vi "Set VRISE.vi"(0 "VISA resource name":refnum<visa-resource-name>, 2 "cluster":cluster{bool, bool, bool, bool}, 5 "error in (no error)":errorcluster) -> (14 "VISA resource name out":refnum<visa-resource-name>, 15 "concatenated string":string, 18 "?":T1 {"Channel 1" format="%#_6e"; "Channel 2" format="%#_6e"; "Channel 3" format="%#_6e"; "Channel 4" format="%#_6e"}, 19 "error out":errorcluster)   [LabVIEW 2018]
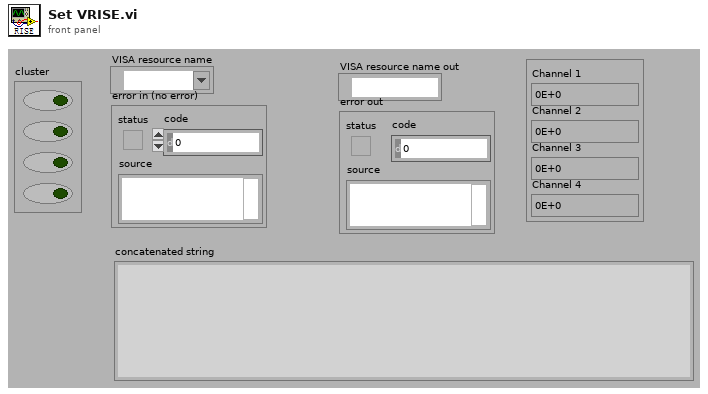
[diagram p1: front panel]
types:
  T1 = cluster{"Channel 1":dbl, "Channel 2":dbl, "Channel 3":dbl, "Channel 4":dbl}
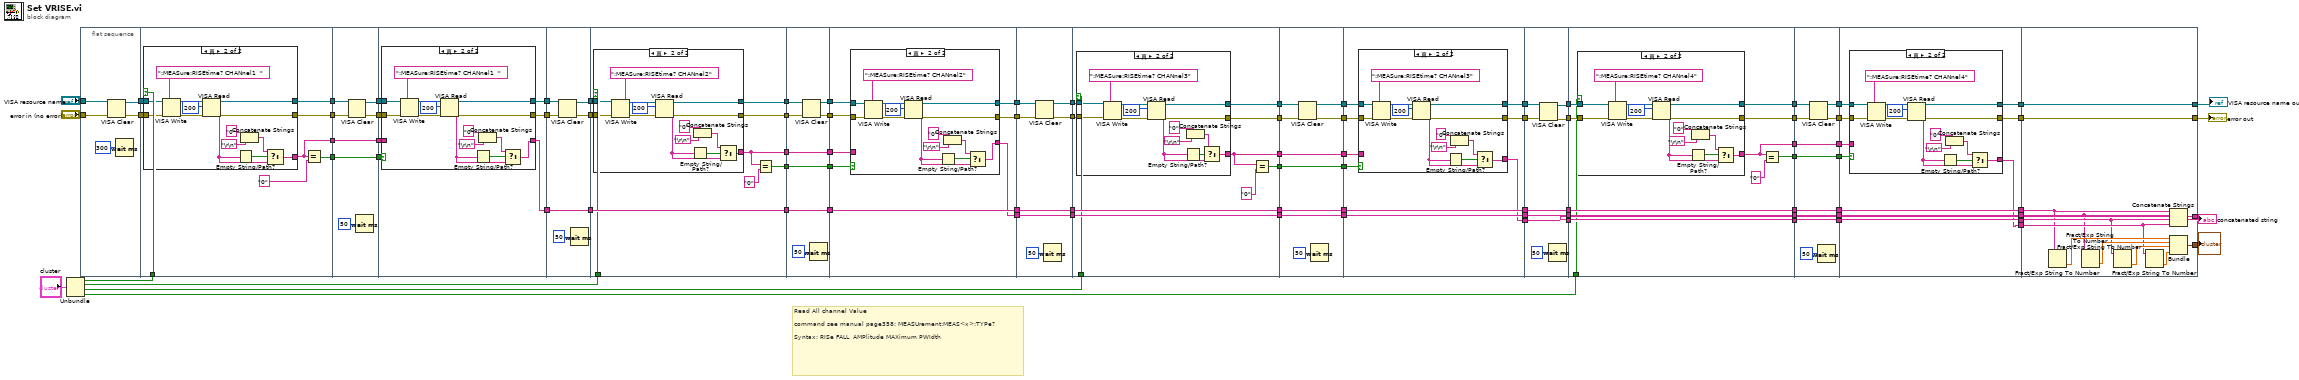
[diagram p0: block diagram]
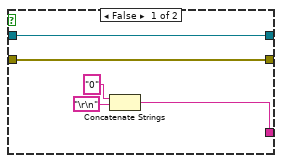
[diagram p2: hidden frame]
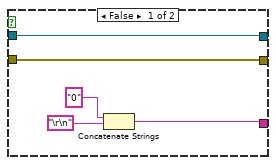
[diagram p4: hidden frame]
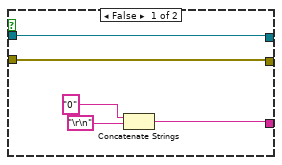
[diagram p6: hidden frame]
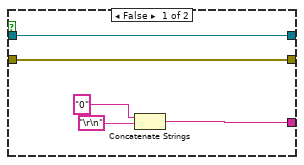
[diagram p8: hidden frame]
diagram:
  # "Read All channel Value\n\ncommand see manual page358: MEASUrement:MEAS<x>:TYPe?\n\nSyntax: RISe FALL  AMPlitude MAXimum PWIdth"
  n1 = Unbundle("cluster") -> (w85:bool, w86:bool, w84:bool, w83:bool)
  n2 = flat-sequence {
    tunnel: [w92] -> w76
    tunnel: [w91] -> w75
    tunnel: "VISA resource name" -> [w89]
    tunnel: "error in (no error)" -> [w88]
    tunnel: w85 -> [w98]
    tunnel: w76 -> [w100]
    tunnel: w75 -> [w99]
    tunnel: [w96] -> w71
    tunnel: [w95] -> w69
    tunnel: [w94] -> w55
    tunnel: [w93] -> w54
    tunnel: [w122] -> w73
    tunnel: [w120] -> w72
    tunnel: w71 -> [w126]
    tunnel: [w126] -> w70
    tunnel: w69 -> [w125]
    tunnel: [w125] -> w68
    tunnel: w55 -> [w123]
    tunnel: w54 -> [w121]
    tunnel: [w127] -> w67
    tunnel: w73 -> [w133]
    tunnel: [w131] -> w65
    tunnel: w72 -> [w132]
    tunnel: [w130] -> w63
    tunnel: w70 -> [w129]
    tunnel: w68 -> [w128]
    tunnel: w67 -> [w156]
    tunnel: [w156] -> w66
    tunnel: w65 -> [w154]
    tunnel: [w153] -> w64
    tunnel: w63 -> [w151]
    tunnel: [w152] -> w1
    tunnel: [w165] -> w74
    tunnel: w66 -> [w165]
    tunnel: w64 -> [w164]
    tunnel: w86 -> [w162]
    tunnel: [w161] -> w62
    tunnel: [w159] -> w56
    tunnel: [w158] -> w53
    tunnel: [w157] -> w52
    tunnel: w1 -> [w163]
    tunnel: w74 -> [w192]
    tunnel: [w192] -> w61
    tunnel: [w186] -> w60
    tunnel: [w185] -> w59
    tunnel: w62 -> [w190]
    tunnel: [w190] -> w58
    tunnel: [w189] -> w57
    tunnel: w56 -> [w189]
    tunnel: w53 -> [w188]
    tunnel: w52 -> [w187]
    tunnel: w61 -> [w200]
    tunnel: [w200] -> w51
    tunnel: [w194] -> w49
    tunnel: w60 -> [w199]
    tunnel: [w197] -> w47
    tunnel: w59 -> [w198]
    tunnel: [w196] -> w45
    tunnel: w58 -> [w195]
    tunnel: w57 -> [w193]
    tunnel: w51 -> [w224]
    tunnel: [w224] -> w50
    tunnel: w49 -> [w223]
    tunnel: [w223] -> w48
    tunnel: w47 -> [w221]
    tunnel: [w220] -> w46
    tunnel: w45 -> [w218]
    tunnel: [w219] -> w44
    tunnel: [w234] -> w43
    tunnel: w50 -> [w234]
    tunnel: [w233] -> w41
    tunnel: w48 -> [w233]
    tunnel: w46 -> [w232]
    tunnel: w44 -> [w231]
    tunnel: w84 -> [w230]
    tunnel: [w228] -> w39
    tunnel: [w227] -> w38
    tunnel: [w226] -> w34
    tunnel: [w225] -> w32
    tunnel: w43 -> [w262]
    tunnel: [w262] -> w42
    tunnel: w41 -> [w261]
    tunnel: [w261] -> w40
    tunnel: w39 -> [w259]
    tunnel: w38 -> [w258]
    tunnel: [w257] -> w37
    tunnel: [w256] -> w36
    tunnel: [w255] -> w35
    tunnel: w34 -> [w255]
    tunnel: [w254] -> w33
    tunnel: w32 -> [w254]
    tunnel: w42 -> [w271]
    tunnel: [w271] -> w31
    tunnel: w40 -> [w270]
    tunnel: [w270] -> w29
    tunnel: [w266] -> w27
    tunnel: w37 -> [w269]
    tunnel: w36 -> [w268]
    tunnel: w35 -> [w267]
    tunnel: w33 -> [w265]
    tunnel: [w264] -> w23
    tunnel: [w263] -> w22
    tunnel: w31 -> [w296]
    tunnel: [w296] -> w30
    tunnel: w29 -> [w295]
    tunnel: [w295] -> w28
    tunnel: w27 -> [w294]
    tunnel: [w294] -> w26
    tunnel: [w291] -> w25
    tunnel: [w289] -> w24
    tunnel: w23 -> [w292]
    tunnel: w22 -> [w290]
    tunnel: [w307] -> w21
    tunnel: w30 -> [w307]
    tunnel: [w306] -> w20
    tunnel: w28 -> [w306]
    tunnel: [w305] -> w19
    tunnel: w26 -> [w305]
    tunnel: w25 -> [w304]
    tunnel: w24 -> [w303]
    tunnel: w83 -> [w302]
    tunnel: [w300] -> w18
    tunnel: [w301] -> w8
    tunnel: [w298] -> w4
    tunnel: [w297] -> w2
    tunnel: w21 -> [w336]
    tunnel: [w336] -> w17
    tunnel: w20 -> [w335]
    tunnel: [w335] -> w15
    tunnel: w19 -> [w334]
    tunnel: [w334] -> w13
    tunnel: w18 -> [w331]
    tunnel: w8 -> [w332]
    tunnel: [w330] -> w7
    tunnel: [w329] -> w6
    tunnel: [w328] -> w5
    tunnel: w4 -> [w328]
    tunnel: [w327] -> w3
    tunnel: w2 -> [w327]
    tunnel: w17 -> [w346]
    tunnel: [w346] -> w16
    tunnel: w15 -> [w345]
    tunnel: [w345] -> w14
    tunnel: w13 -> [w344]
    tunnel: [w344] -> w12
    tunnel: [w339] -> w11
    tunnel: [w341] -> w10
    tunnel: [w340] -> w9
    tunnel: w7 -> [w343]
    tunnel: w6 -> [w342]
    tunnel: w5 -> [w338]
    tunnel: w3 -> [w337]
    tunnel: w16 -> [w366]
    tunnel: w14 -> [w367]
    tunnel: w12 -> [w368]
    tunnel: w11 -> [w369]
    tunnel: [w371] -> w87
    tunnel: [w370] -> w79
    tunnel: [w365] -> w78
    tunnel: w10 -> [w365]
    tunnel: w9 -> [w364]
    tunnel: [w364] -> w77
    frame #0 {
      n3 = VISA Clear(VISA resource name=w89, error in (no error)=w88) -> (VISA resource name out=w91:refnum<visa-resource-name>, error out=w92:errorcluster)
      n4 = Wait (ms)(milliseconds to wait=u32 300) -> ()  [unwired: 1 out]
    }
    frame #1 {
      n5 = case shown="真" w98 {
        tunnel: [w101 w106] -> w95
        tunnel: [w105 w115] -> w94
        tunnel: [w104 w114] -> w93
        tunnel: w100 -> [w104 w113]
        tunnel: w99 -> [w105 w112]
        frame False {
          n6 = Concatenate Strings("0" ("write buffer"), "\r\n") -> (w101:string)
        }
        frame True {
          n7 = VISA Write(VISA resource name=w112, write buffer=":MEASure:RISEtime? CHANnel1  ", error in (no error)=w113) -> (VISA resource name out=w117:refnum<visa-resource-name>, error out=w118:errorcluster)  [unwired: 1 out]
          n8 = VISA Read(VISA resource name=w117, byte count=u32 200, error in (no error)=w118) -> (VISA resource name out=w115:refnum<visa-resource-name>, read buffer=w107:string, error out=w114:errorcluster)  [unwired: 1 out]
          n9 = Empty String/Path?(string/path=w107) -> (empty?=w111:bool)
          n10 = Concatenate Strings("0" ("write buffer"), "\r\n") -> (w108:string)
          n11 = Select(t=w108, s=w111, f=w107) -> (s? t:f=w106:string)
        }
      }
      n12 = Equal?(x=w95, y="0" ("write buffer")) -> (x = y?=w96:bool)
    }
    frame #2 {
      n13 = VISA Clear(VISA resource name=w123, error in (no error)=w121) -> (VISA resource name out=w122:refnum<visa-resource-name>, error out=w120:errorcluster)
      n14 = Wait (ms)(milliseconds to wait=u32 50) -> ()  [unwired: 1 out]
    }
    frame #3 {
      n15 = case shown="真" w129 {
        tunnel: [w136 w146] -> w131
        tunnel: [w135 w145] -> w130
        tunnel: w132 -> [w135 w144]
        tunnel: w133 -> [w136 w143]
        tunnel: [w134 w137] -> w127
        tunnel: w128 -> [w134 _]
        frame False {
        }
        frame True {
          n16 = VISA Write(VISA resource name=w143, write buffer=":MEASure:RISEtime? CHANnel1  ", error in (no error)=w144) -> (VISA resource name out=w148:refnum<visa-resource-name>, error out=w149:errorcluster)  [unwired: 1 out]
          n17 = VISA Read(VISA resource name=w148, byte count=u32 200, error in (no error)=w149) -> (VISA resource name out=w146:refnum<visa-resource-name>, read buffer=w138:string, error out=w145:errorcluster)  [unwired: 1 out]
          n18 = Empty String/Path?(string/path=w138) -> (empty?=w142:bool)
          n19 = Concatenate Strings("0" ("write buffer"), "\r\n") -> (w139:string)
          n20 = Select(t=w139, s=w142, f=w138) -> (s? t:f=w137:string)
        }
      }
    }
    frame #4 {
      n21 = VISA Clear(VISA resource name=w154, error in (no error)=w151) -> (VISA resource name out=w153:refnum<visa-resource-name>, error out=w152:errorcluster)
      n22 = Wait (ms)(milliseconds to wait=u32 50) -> ()  [unwired: 1 out]
    }
    frame #5 {
      n23 = case shown="真" w162 {
        tunnel: [w166 w171] -> w161
        tunnel: w164 -> [w170 w180]
        tunnel: [w170 w179] -> w158
        tunnel: w163 -> [w169 w178]
        tunnel: [w169 w177] -> w157
        frame False {
          n24 = Concatenate Strings("0" ("write buffer"), "\r\n") -> (w166:string)
        }
        frame True {
          n25 = VISA Write(VISA resource name=w180, write buffer=":MEASure:RISEtime? CHANnel2", error in (no error)=w178) -> (VISA resource name out=w182:refnum<visa-resource-name>, error out=w183:errorcluster)  [unwired: 1 out]
          n26 = VISA Read(VISA resource name=w182, byte count=u32 200, error in (no error)=w183) -> (VISA resource name out=w179:refnum<visa-resource-name>, read buffer=w172:string, error out=w177:errorcluster)  [unwired: 1 out]
          n27 = Empty String/Path?(string/path=w172) -> (empty?=w176:bool)
          n28 = Concatenate Strings("0" ("write buffer"), "\r\n") -> (w173:string)
          n29 = Select(t=w173, s=w176, f=w172) -> (s? t:f=w171:string)
        }
      }
      n30 = Equal?(x=w161, y="0" ("write buffer")) -> (x = y?=w159:bool)
    }
    frame #6 {
      n31 = VISA Clear(VISA resource name=w188, error in (no error)=w187) -> (VISA resource name out=w186:refnum<visa-resource-name>, error out=w185:errorcluster)
      n32 = Wait (ms)(milliseconds to wait=u32 50) -> ()  [unwired: 1 out]
    }
    frame #7 {
      n33 = case shown="真" w193 {
        tunnel: [w203 w213] -> w197
        tunnel: [w202 w212] -> w196
        tunnel: w198 -> [w202 w211]
        tunnel: w199 -> [w203 w210]
        tunnel: [w201 w204] -> w194
        tunnel: w195 -> [w201 _]
        frame False {
        }
        frame True {
          n34 = VISA Write(VISA resource name=w210, write buffer=":MEASure:RISEtime? CHANnel2", error in (no error)=w211) -> (VISA resource name out=w215:refnum<visa-resource-name>, error out=w216:errorcluster)  [unwired: 1 out]
          n35 = VISA Read(VISA resource name=w215, byte count=u32 200, error in (no error)=w216) -> (VISA resource name out=w213:refnum<visa-resource-name>, read buffer=w205:string, error out=w212:errorcluster)  [unwired: 1 out]
          n36 = Empty String/Path?(string/path=w205) -> (empty?=w209:bool)
          n37 = Concatenate Strings("0" ("write buffer"), "\r\n") -> (w206:string)
          n38 = Select(t=w206, s=w209, f=w205) -> (s? t:f=w204:string)
        }
      }
    }
    frame #8 {
      n39 = VISA Clear(VISA resource name=w221, error in (no error)=w218) -> (VISA resource name out=w220:refnum<visa-resource-name>, error out=w219:errorcluster)
      n40 = Wait (ms)(milliseconds to wait=u32 50) -> ()  [unwired: 1 out]
    }
    frame #9 {
      n41 = case shown="真" w230 {
        tunnel: [w235 w240] -> w225
        tunnel: w232 -> [w239 w249]
        tunnel: [w239 w248] -> w228
        tunnel: w231 -> [w238 w247]
        tunnel: [w238 w246] -> w227
        frame False {
          n42 = Concatenate Strings("0" ("write buffer"), "\r\n") -> (w235:string)
        }
        frame True {
          n43 = VISA Write(VISA resource name=w249, write buffer=":MEASure:RISEtime? CHANnel3", error in (no error)=w247) -> (VISA resource name out=w251:refnum<visa-resource-name>, error out=w252:errorcluster)  [unwired: 1 out]
          n44 = VISA Read(VISA resource name=w251, byte count=u32 200, error in (no error)=w252) -> (VISA resource name out=w248:refnum<visa-resource-name>, read buffer=w241:string, error out=w246:errorcluster)  [unwired: 1 out]
          n45 = Empty String/Path?(string/path=w241) -> (empty?=w245:bool)
          n46 = Concatenate Strings("0" ("write buffer"), "\r\n") -> (w242:string)
          n47 = Select(t=w242, s=w245, f=w241) -> (s? t:f=w240:string)
        }
      }
      n48 = Equal?(x=w225, y="0" ("write buffer")) -> (x = y?=w226:bool)
    }
    frame #10 {
      n49 = VISA Clear(VISA resource name=w259, error in (no error)=w258) -> (VISA resource name out=w257:refnum<visa-resource-name>, error out=w256:errorcluster)
      n50 = Wait (ms)(milliseconds to wait=u32 50) -> ()  [unwired: 1 out]
    }
    frame #11 {
      n51 = case shown="真" w267 {
        tunnel: [w274 w284] -> w264
        tunnel: [w273 w283] -> w263
        tunnel: w268 -> [w273 w282]
        tunnel: w269 -> [w274 w281]
        tunnel: [w272 w275] -> w266
        tunnel: w265 -> [w272 _]
        frame False {
        }
        frame True {
          n52 = VISA Write(VISA resource name=w281, write buffer=":MEASure:RISEtime? CHANnel3", error in (no error)=w282) -> (VISA resource name out=w286:refnum<visa-resource-name>, error out=w287:errorcluster)  [unwired: 1 out]
          n53 = VISA Read(VISA resource name=w286, byte count=u32 200, error in (no error)=w287) -> (VISA resource name out=w284:refnum<visa-resource-name>, read buffer=w276:string, error out=w283:errorcluster)  [unwired: 1 out]
          n54 = Empty String/Path?(string/path=w276) -> (empty?=w280:bool)
          n55 = Concatenate Strings("0" ("write buffer"), "\r\n") -> (w277:string)
          n56 = Select(t=w277, s=w280, f=w276) -> (s? t:f=w275:string)
        }
      }
    }
    frame #12 {
      n57 = VISA Clear(VISA resource name=w292, error in (no error)=w290) -> (VISA resource name out=w291:refnum<visa-resource-name>, error out=w289:errorcluster)
      n58 = Wait (ms)(milliseconds to wait=u32 50) -> ()  [unwired: 1 out]
    }
    frame #13 {
      n59 = case shown="真" w302 {
        tunnel: [w308 w313] -> w297
        tunnel: w304 -> [w312 w322]
        tunnel: [w312 w321] -> w301
        tunnel: [w311 w320] -> w300
        tunnel: w303 -> [w311 w319]
        frame False {
          n60 = Concatenate Strings("0" ("write buffer"), "\r\n") -> (w308:string)
        }
        frame True {
          n61 = VISA Write(VISA resource name=w322, write buffer=":MEASure:RISEtime? CHANnel4", error in (no error)=w319) -> (VISA resource name out=w324:refnum<visa-resource-name>, error out=w325:errorcluster)  [unwired: 1 out]
          n62 = VISA Read(VISA resource name=w324, byte count=u32 200, error in (no error)=w325) -> (VISA resource name out=w321:refnum<visa-resource-name>, read buffer=w314:string, error out=w320:errorcluster)  [unwired: 1 out]
          n63 = Empty String/Path?(string/path=w314) -> (empty?=w318:bool)
          n64 = Concatenate Strings("0" ("write buffer"), "\r\n") -> (w315:string)
          n65 = Select(t=w315, s=w318, f=w314) -> (s? t:f=w313:string)
        }
      }
      n66 = Equal?(x=w297, y="0" ("write buffer")) -> (x = y?=w298:bool)
    }
    frame #14 {
      n67 = VISA Clear(VISA resource name=w332, error in (no error)=w331) -> (VISA resource name out=w330:refnum<visa-resource-name>, error out=w329:errorcluster)
      n68 = Wait (ms)(milliseconds to wait=u32 50) -> ()  [unwired: 1 out]
    }
    frame #15 {
      n69 = case shown="真" w338 {
        tunnel: [w349 w359] -> w341
        tunnel: [w348 w358] -> w340
        tunnel: w342 -> [w348 w357]
        tunnel: w343 -> [w349 w356]
        tunnel: [w347 w350] -> w339
        tunnel: w337 -> [w347 _]
        frame False {
        }
        frame True {
          n70 = VISA Write(VISA resource name=w356, write buffer=":MEASure:RISEtime? CHANnel4", error in (no error)=w357) -> (VISA resource name out=w361:refnum<visa-resource-name>, error out=w362:errorcluster)  [unwired: 1 out]
          n71 = VISA Read(VISA resource name=w361, byte count=u32 200, error in (no error)=w362) -> (VISA resource name out=w359:refnum<visa-resource-name>, read buffer=w351:string, error out=w358:errorcluster)  [unwired: 1 out]
          n72 = Empty String/Path?(string/path=w351) -> (empty?=w355:bool)
          n73 = Concatenate Strings("0" ("write buffer"), "\r\n") -> (w352:string)
          n74 = Select(t=w352, s=w355, f=w351) -> (s? t:f=w350:string)
        }
      }
    }
    frame #16 {
      n75 = Fract/Exp String To Number(string=w366) -> (number=w372:dbl)  [unwired: 3 in, 1 out]
      n76 = Fract/Exp String To Number(string=w367) -> (number=w375:dbl)  [unwired: 3 in, 1 out]
      n77 = Fract/Exp String To Number(string=w368) -> (number=w374:dbl)  [unwired: 3 in, 1 out]
      n78 = Fract/Exp String To Number(string=w369) -> (number=w373:dbl)  [unwired: 3 in, 1 out]
      n79 = Concatenate Strings(w366, w367, w368, w369) -> (w370:string)
      n80 = Bundle(w372, w375, w374, w373) -> (w371:cluster{dbl, dbl, dbl, dbl})  [unwired: 1 in]
    }
  }
  "VISA resource name out" <- w78
  "error out" <- w77
  "concatenated string" <- w79
  "?" <- w87
